vi "Config File FGV.vi"(7 "Amount Deposited In":string, 8 "error in (no error)":errorcluster, 9 "Column(0)":i32, 10 "Row(0)":i32, 11 "ini File Operation":T1) -> (0 "error out":errorcluster, 1 "Transaction Success?":bool, 2 "Change Returned Out":string, 3 "Vending Panel Out":T2[][](array[typedef]), 5 "Amount Deposited Out":string)   [LabVIEW 2020]
doc: "This VI can Open, Read, modifies, Updates and Closes the ini File."
uses:
  Controller/Product Select.ctl
  Controller/ini File Operation.ctl
  <vilib>/Utility/config.llb/Read Key (String).vi
  <vilib>/Utility/config.llb/Read Key (I32).vi
  <vilib>/Utility/config.llb/Write Key (String).vi
  <vilib>/Utility/config.llb/NI_LVConfig.lvlib
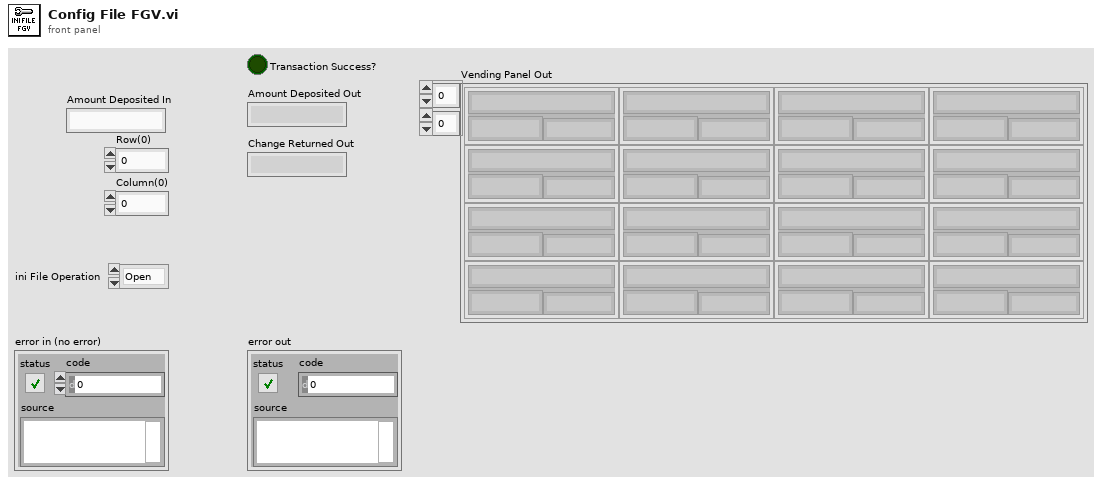
[diagram p1: front panel]
types:
  T1 = typedef "ini File Operation.ctl" = enum16{"Open", "Read", "Check", "Update", "Close"}
  T2 = typedef "Product Select.ctl" = cluster{"Product Name":string, "Product Cost":string, "Inventory":string}
  T3 = typedef "NI_LVConfig.lvlib/Config Data RefNum.ctl" = refnum<k1>
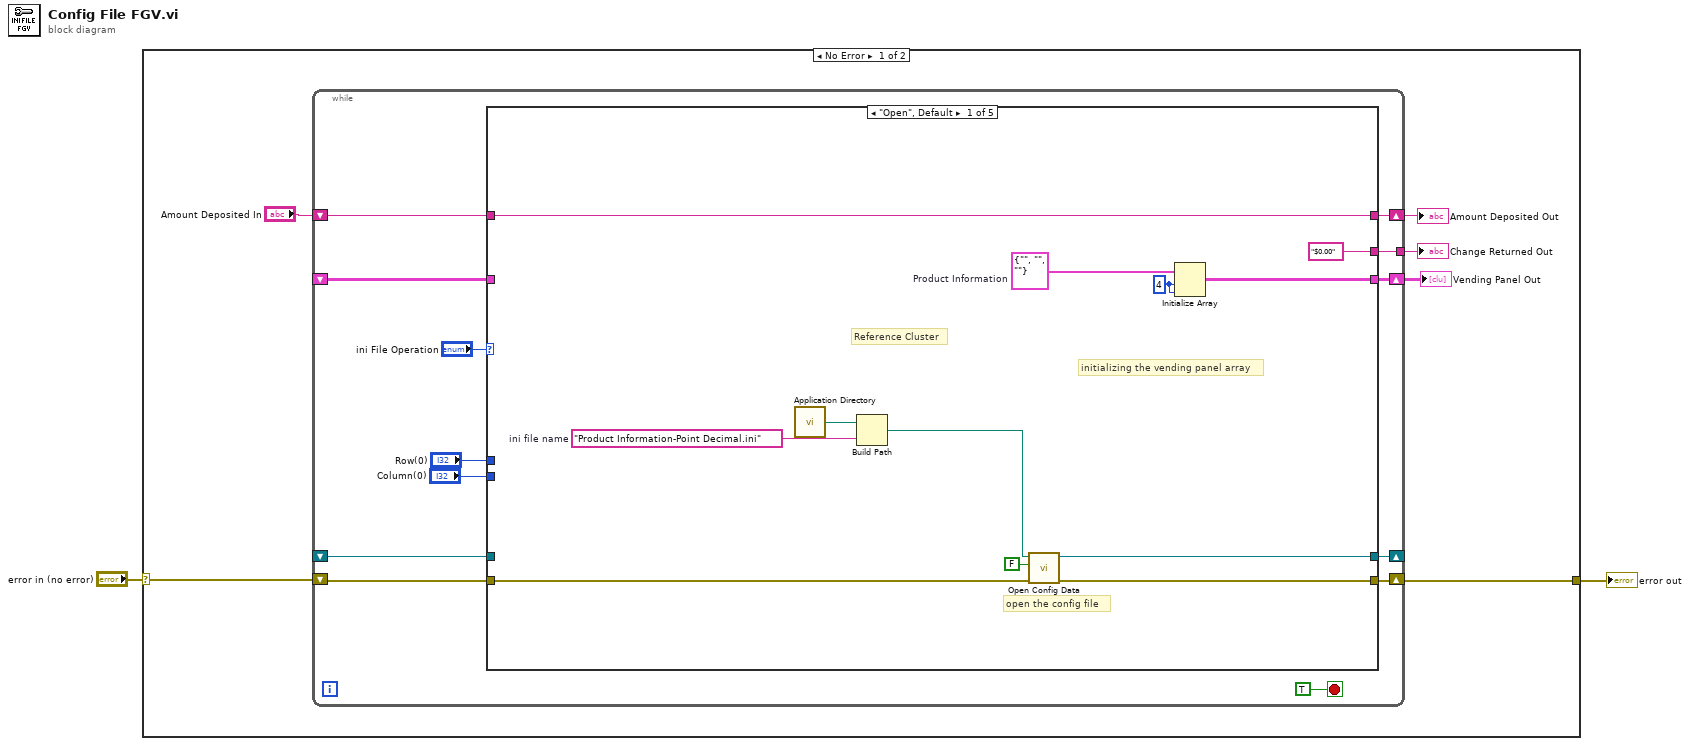
[diagram p0: block diagram]
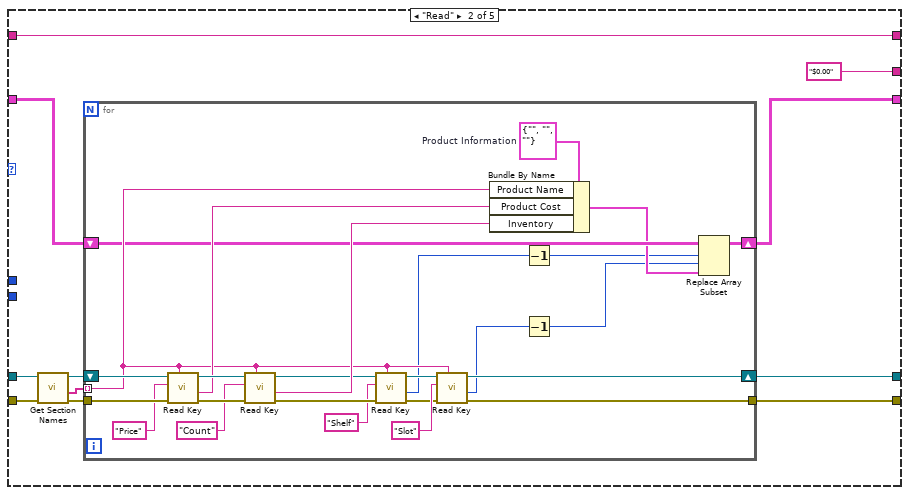
[diagram p2: hidden frame]
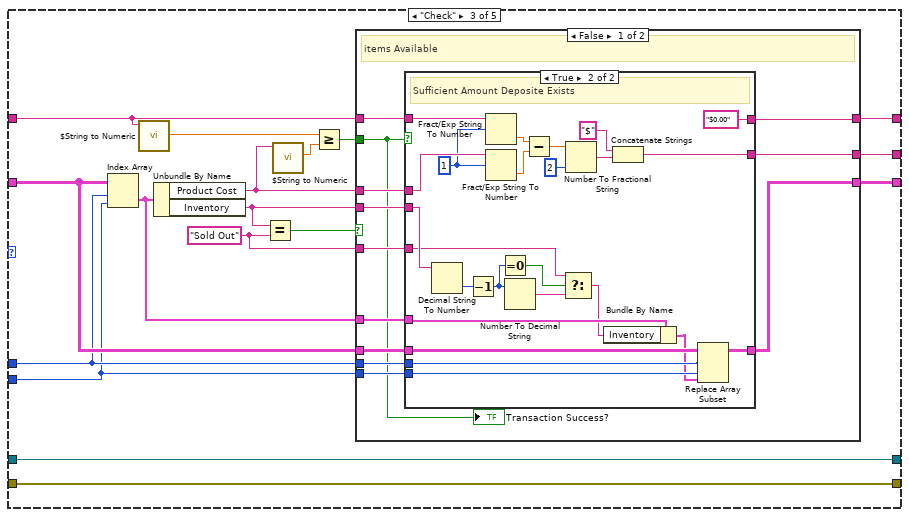
[diagram p3: hidden frame]
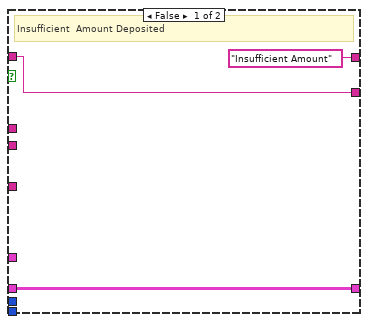
[diagram p4: hidden frame]
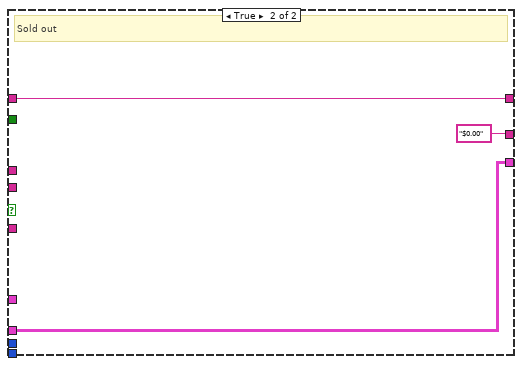
[diagram p5: hidden frame]
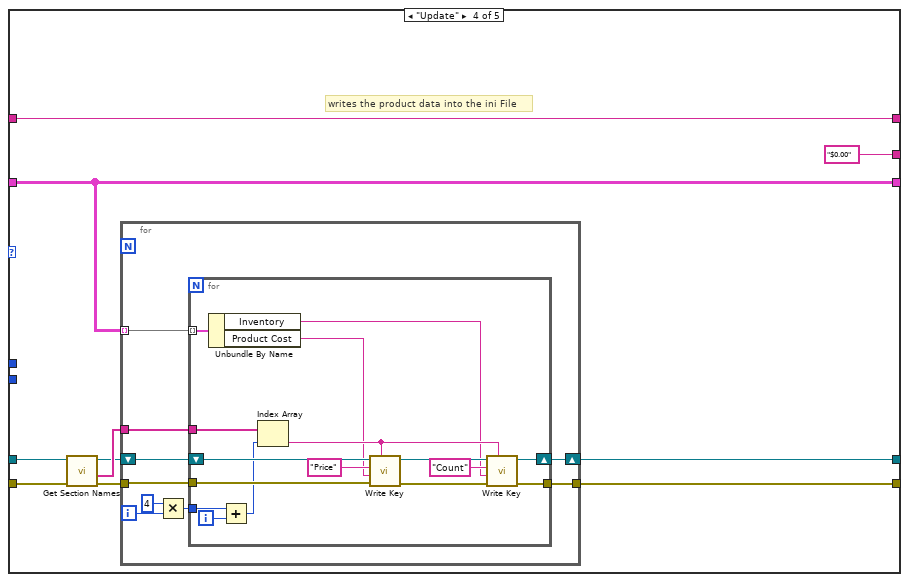
[diagram p6: hidden frame]
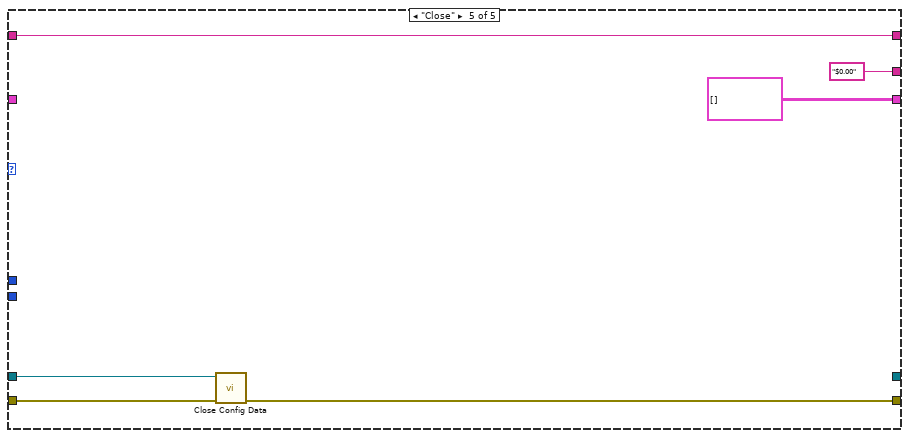
[diagram p7: hidden frame]
diagram:
  n1 = case shown="No Error" "error in (no error)" {
    selector: "error in (no error)" -> [w7 w170]
    tunnel: [w8 w170] -> w2
    frame No Error {
      n2 = while {
        shift-right: [w21] -> w6
        shift-left: _ -> [w20]
        shift-right: [w18] -> _
        shift-left: _ -> [w17]
        shift-right: [w19] -> w8
        shift-left: w7 -> [w15]
        tunnel: [w11] -> w5
        shift-right: [w9] -> w3
        shift-left: "Amount Deposited In" -> [w10]
        stop <- TRUE stop-if-true
        n3 = case shown="\"Open\", Default" "ini File Operation" {
          tunnel: [w24 w44 w77 w130 T2[][] [] ("Vending Panel IN")] -> w21
          tunnel: w20 -> [_ w43 w80 w130 _]
          tunnel: [w31 w42 w84 w132 w167] -> w19
          tunnel: [w30 w41 w82 w131 _] -> w18
          tunnel: w15 -> [w33 w38 w84 w136 w169]
          tunnel: w17 -> [_ w37 w82 w138 w168]
          tunnel: "Row(0)" -> [_ _ w79 _ _]
          tunnel: "Column(0)" -> [_ _ w78 _ _]
          tunnel: w10 -> [w23 w36 w75 w137 w165]
          tunnel: ["$0.00" "$0.00" w83 "$0.00" "$0.00"] -> w11
          tunnel: [w23 w36 w76 w137 w165] -> w9
          frame "Open", Default {
            w25 = 4 ("dimension size")
            w26 = T2 {"Product Name"="", "Product Cost"="", "Inventory"=""}  # Product Information
            w29 = "Product Information-Point Decimal.ini"  # ini file name
            # "Reference Cluster"
            # "open the config file"
            # "initializing the vending panel array"
            n4 = call <vilib>:"Application Directory.vi"() -> ("Application Directory"=w27:path)
            n5 = Build Path(base path=w27, name or relative path=w29) -> (appended path=w28:path)
            n6 = call <vilib>:"Open Config Data.vi"("error in (no error)"=w33, "create file if necessary (T)"=FALSE, "configuration file path"=w28) -> ("error out"=w31:errorcluster, "refnum"=w30:T3)  [unwired: 6 in, 1 out]
            n7 = Initialize Array(w26, w25, w25) -> (w24:T2[][])
          }
          frame "Read" {
            n8 = call <vilib>:"Get Section Names.vi"("error in (no error)"=w38, "refnum"=w37) -> ("error out"=w40:errorcluster, "section names"=w35:string[], "refnum out"=w39:T3)  [unwired: 7 in]
            n9 = for {
              tunnel: w35 -> [w53] mode=indexing
              tunnel: w40 -> [w68]
              tunnel: [w63] -> w42
              shift-right: [w64] -> w41
              shift-left: w39 -> [w69]
              shift-right: [w50] -> w44
              shift-left: w43 -> [w52]
              w49 = T2 {"Product Name"="", "Product Cost"="", "Inventory"=""}  # Product Information
              n10 = call-poly <vilib>:"Read Key.vi"("section"=w53, "error in (no error)"=w68, "key"="Price", "refnum"=w69) -> ("error out"=w65:errorcluster, "value"=w62:string, "refnum out"=w67:T3)  [unwired: 4 in, 1 out]
              n11 = call-poly <vilib>:"Read Key.vi"("section"=w53, "error in (no error)"=w65, "key"="Count", "refnum"=w67) -> ("error out"=w57:errorcluster, "value"=w61:string, "refnum out"=w58:T3)  [unwired: 4 in, 1 out]
              n12 = call-poly <vilib>:"Read Key.vi"("section"=w53, "error in (no error)"=w57, "key"="Shelf", "refnum"=w58) -> ("error out"=w55:errorcluster, "value"=w51:i32, "refnum out"=w56:T3)  [unwired: 4 in, 1 out]
              n13 = call-poly <vilib>:"Read Key.vi"("section"=w53, "error in (no error)"=w55, "key"="Slot", "refnum"=w56) -> ("error out"=w63:errorcluster, "value"=w48:i32, "refnum out"=w64:T3)  [unwired: 4 in, 1 out]
              n14 = Bundle By Name(cluster=w49, "Product Name"=w53, "Product Cost"=w62, "Inventory"=w61) -> (w47:T2)
              n15 = Decrement(x=w51) -> (x-1=w46:i32)
              n16 = Decrement(x=w48) -> (x-1=w45:i32)
              n17 = Replace Array Subset(array=w52, new element=w47, index (row)=w46, index (col)=w45) -> (w50:T2[][])
            }
          }
          frame "Check" {
            w85 = "Sold Out" ("y")
            n18 = Index Array(array=w80, index (row)=w79, index (col)=w78) -> (element=w81:T2)
            n19 = call "$String to Numeric.vi"("Amount Deposited In"=w75) -> ("Amount"=w73:dbl)  [unwired: 9 in, 1 out]
            n20 = Unbundle By Name(w81) -> ("Product Cost"=w74:string, "Inventory"=w86:string)
            n21 = Equal?(x=w86, y=w85) -> (x = y?=w71:bool)
            n22 = call "$String to Numeric.vi"("Amount Deposited In"=w74) -> ("Amount"=w72:dbl)  [unwired: 9 in, 1 out]
            n23 = Greater Or Equal?(x=w73, y=w72) -> (x >= y?=w70:bool)
            n24 = case shown="False" w71 {
              tunnel: w86 -> [w98 _]
              tunnel: w74 -> [w97 _]
              tunnel: w85 -> [w96 _]
              tunnel: w75 -> [w95 w126]
              tunnel: [w94 "$0.00"] -> w83
              tunnel: w81 -> [w93 _]
              tunnel: w80 -> [w92 w127]
              tunnel: w79 -> [w91 _]
              tunnel: w78 -> [w90 _]
              tunnel: [w89 w127] -> w77
              tunnel: [w88 w126] -> w76
              tunnel: w70 -> [w87 _]
              frame False {
                # "items Available"
                n25 = case shown="True" w87 {
                  tunnel: w98 -> [_ w125]
                  tunnel: w97 -> [_ w119]
                  tunnel: w96 -> [_ w122]
                  tunnel: w95 -> [w99 w117]
                  tunnel: [w99 w111] -> w94
                  tunnel: w93 -> [_ w110]
                  tunnel: w92 -> [w101 w108]
                  tunnel: w91 -> [_ w107]
                  tunnel: w90 -> [_ w106]
                  tunnel: [w101 w104] -> w89
                  tunnel: ["Insufficient Amount" ("Amount Deposited In") "$0.00" ("Amount Deposited In")] -> w88
                  frame False {
                    # "Insufficient  Amount Deposited"
                  }
                  frame True {
                    w118 = 1 ("offset")
                    # "Sufficient Amount Deposite Exists"
                    n26 = Decimal String To Number(string=w125) -> (number=w124:i32)  [unwired: 2 in, 1 out]
                    n27 = Decrement(x=w124) -> (x-1=w121:i32)
                    n28 = Fract/Exp String To Number(string=w117, offset=w118) -> (number=w116:dbl)  [unwired: 2 in, 1 out]
                    n29 = Fract/Exp String To Number(string=w119, offset=w118) -> (number=w115:dbl)  [unwired: 2 in, 1 out]
                    n30 = Equal To 0?(x=w121) -> (x = 0?=w123:bool)
                    n31 = Number To Decimal String(number=w121) -> (decimal integer string=w120:string)  [unwired: 1 in]
                    n32 = Subtract(x=w116, y=w115) -> (x-y=w114:dbl)
                    n33 = Select(t=w122, s=w123, f=w120) -> (s? t:f=w109:string)
                    n34 = Number To Fractional String(number=w114, precision (6)=i16 2 ("width (-)")) -> (F-format string=w113:string)  [unwired: 2 in]
                    n35 = Bundle By Name(cluster=w110, "Inventory"=w109) -> (w105:T2)
                    n36 = Concatenate Strings("$" ("string"), w113) -> (w111:string)
                    n37 = Replace Array Subset(array=w108, new element=w105, index (row)=w107, index (col)=w106) -> (w104:T2[][])
                  }
                }
                "Transaction Success?" <- w87
              }
              frame True {
                # "Sold out"
              }
            }
          }
          frame "Update" {
            # "writes the product data into the ini File"
            n38 = call <vilib>:"Get Section Names.vi"("error in (no error)"=w136, "refnum"=w138) -> ("error out"=w135:errorcluster, "section names"=w134:string[], "refnum out"=w133:T3)  [unwired: 7 in]
            n39 = for {
              tunnel: w135 -> [w146]
              tunnel: w134 -> [w145]
              tunnel: w130 -> [w143] mode=indexing
              shift-right: [w140] -> w131
              shift-left: w133 -> [w147]
              tunnel: [w139] -> w132
              i -> [w144]
              n40 = Multiply(x=4, y=w144) -> (x*y=w141:i32)
              n41 = for {
                tunnel: w146 -> [w161]
                tunnel: w143 -> [w152] mode=indexing
                tunnel: w145 -> [w155]
                tunnel: w141 -> [w156]
                shift-right: [w150] -> w140
                shift-left: w147 -> [w162]
                tunnel: [w149] -> w139
                i -> [w157]
                n42 = Unbundle By Name(w152) -> ("Inventory"=w151:string, "Product Cost"=w148:string)
                n43 = Add(x=w156, y=w157) -> (x+y=w154:i32)
                n44 = Index Array(array=w155, index=w154) -> (element=w153:string)
                n45 = call-poly <vilib>:"Write Key.vi"("section"=w153, "error in (no error)"=w161, "value"=w148, "key"="Price", "refnum"=w162) -> ("error out"=w163:errorcluster, "refnum out"=w160:T3)  [unwired: 4 in, 1 out]
                n46 = call-poly <vilib>:"Write Key.vi"("section"=w153, "error in (no error)"=w163, "value"=w151, "key"="Count", "refnum"=w160) -> ("error out"=w149:errorcluster, "refnum out"=w150:T3)  [unwired: 4 in, 1 out]
              }
            }
          }
          frame "Close" {
            n47 = call <vilib>:"Close Config Data.vi"("error in (no error)"=w169, "refnum"=w168) -> ("error out"=w167:errorcluster)  [unwired: 8 in, 1 out]
          }
        }
      }
      "Vending Panel Out" <- w6
      "Change Returned Out" <- w5
      "Amount Deposited Out" <- w3
    }
    frame Error {
    }
  }
  "error out" <- w2
